vi "TouchPanel.setGUIrefs.vi"(0 "register mode (close & register)":enum16{"close & register", "register", "close"}(ring), 7 "Current screen name":string, 11 "error in (no error)":errorcluster) -> (6 "Prev screen VI name":string, 15 "dup of error in":errorcluster)   [LabVIEW 2015]
uses:
  TouchPanel.Global.vi
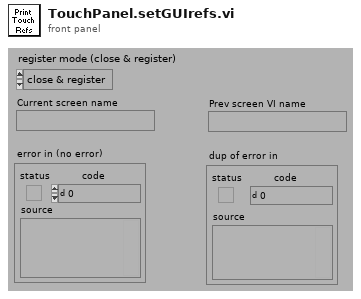
[diagram p1: front panel]
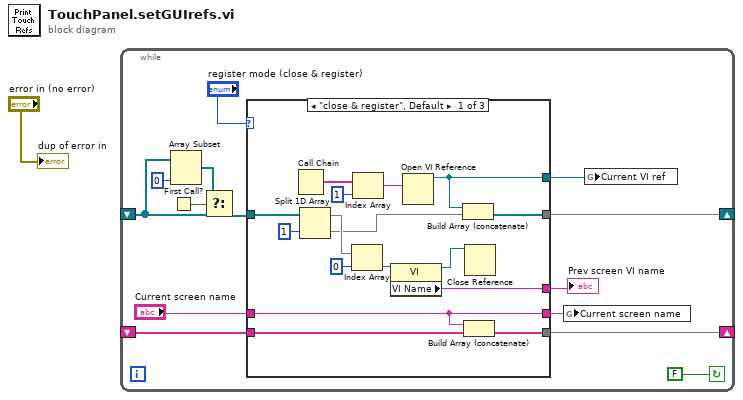
[diagram p0: block diagram]
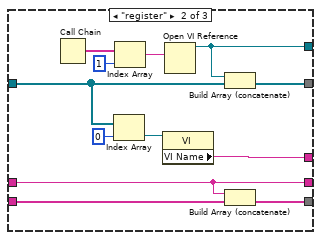
[diagram p2: hidden frame]
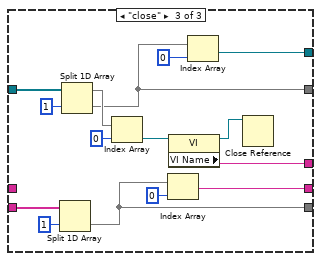
[diagram p3: hidden frame]
diagram:
  n1 = while {
    shift-right: [w14] -> _
    shift-left: _ -> [w9]
    shift-right: [w4] -> _
    shift-left: _ -> [w7]
    stop <- FALSE continue-if-true
    n2 = First Call?() -> (First Call?: T/F=w11:bool)
    n3 = Array Subset(array=w9, length=0) -> (w10:refnum<vi>[])  [unwired: 1 in]
    n4 = Select(t=w10, s=w11, f=w9) -> (s? t:f=w12:refnum<vi>[])
    n5 = case shown="\"close & register\", Default" "register mode (close & register)" {
      tunnel: w12 -> [w31 w35 w58]
      tunnel: [w24 w41 w46] -> w14
      tunnel: w7 -> [w22 w39 w53]
      tunnel: [w20 w38 w51] -> w6
      tunnel: "Current screen name" -> [w20 w38 _]
      tunnel: [w21 w37 w50] -> w4
      tunnel: [w17 w33 w48] -> w3
      tunnel: [w16 w32 w44] -> w2
      frame "close & register", Default {
        n6 = Call Chain() -> (call chain=w26:string[])
        n7 = Split 1D Array(array=w31, index=1) -> (first subarray=w29:refnum<vi>[], second subarray=w25:refnum<vi>[])
        n8 = Index Array(array=w29, index=0) -> (element=w19:refnum<vi>)
        n9 = Index Array(array=w26, index=1) -> (element=w23:string)
        n10 = property class="VI"(reference=w19) -> (reference out=w18:refnum<vi>, "VI Name"=w17:string)  [unwired: 1 in, 1 out]
        n11 = Open VI Reference(vi path=w23) -> (vi reference=w16:refnum<vi>)  [unwired: 1 in, 5 out]
        n12 = Build Array (concatenate)(w16, w25) -> (w24:refnum<vi>[])
        n13 = Build Array (concatenate)(w20, w22) -> (w21:string[])
        n14 = Close Reference(reference=w18) -> ()  [unwired: 1 in, 1 out]
      }
      frame "register" {
        n15 = Call Chain() -> (call chain=w42:string[])
        n16 = Index Array(array=w35, index=0) -> (element=w34:refnum<vi>)
        n17 = Index Array(array=w42, index=1) -> (element=w40:string)
        n18 = property class="VI"(reference=w34) -> ("VI Name"=w33:string)  [unwired: 1 in, 2 out]
        n19 = Open VI Reference(vi path=w40) -> (vi reference=w32:refnum<vi>)  [unwired: 1 in, 5 out]
        n20 = Build Array (concatenate)(w32, w35) -> (w41:refnum<vi>[])
        n21 = Build Array (concatenate)(w38, w39) -> (w37:string[])
      }
      frame "close" {
        n22 = Split 1D Array(array=w53, index=1) -> (second subarray=w50:string[])  [unwired: 1 out]
        n23 = Split 1D Array(array=w58, index=1) -> (first subarray=w56:refnum<vi>[], second subarray=w46:refnum<vi>[])
        n24 = Index Array(array=w56, index=0) -> (element=w47:refnum<vi>)
        n25 = Index Array(array=w50, index=0) -> (element=w51:string)
        n26 = property class="VI"(reference=w47) -> (reference out=w49:refnum<vi>, "VI Name"=w48:string)  [unwired: 1 in, 1 out]
        n27 = Index Array(array=w46, index=0) -> (element=w44:refnum<vi>)
        n28 = Close Reference(reference=w49) -> ()  [unwired: 1 in, 1 out]
      }
    }
    "Prev screen VI name" <- w3
    n29 = global write "TouchPanel.Global.vi" "Current screen name"(w6) -> ()
    n30 = global write "TouchPanel.Global.vi" "Current VI ref"(w2) -> ()
  }
  "dup of error in" <- "error in (no error)"
